vi "SNA Driver Calibration Popup.vi"(8 "error in (no error)":errorcluster, 10 "RequestedCal":string, 11 "Message (\"\")":string) -> (0 "error out":errorcluster)   [LabVIEW 2011]
panel:
  in  "OK":bool
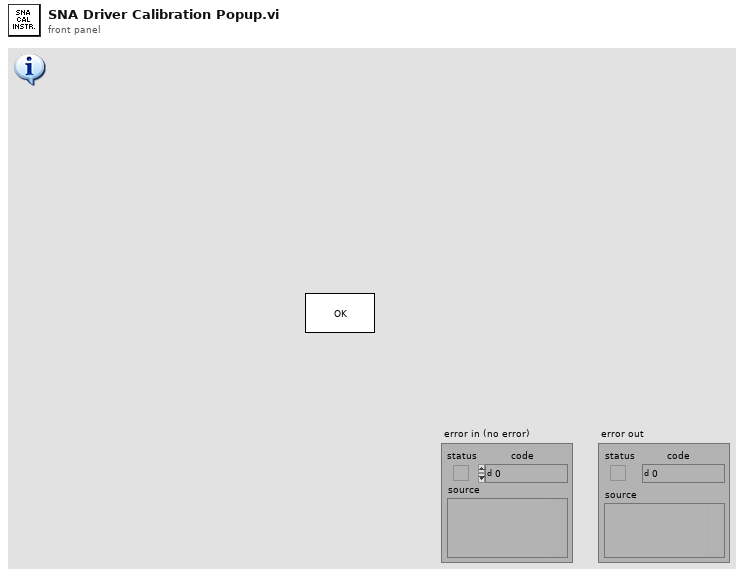
[diagram p1: front panel]
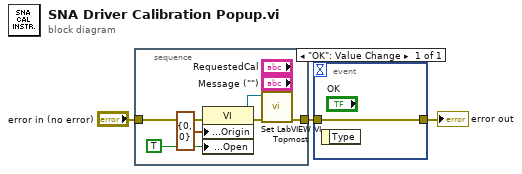
[diagram p0: block diagram]
diagram:
  n1 = stacked-sequence {
    tunnel: "error in (no error)" -> [w9]
    tunnel: [w6] -> w1
    frame #0 {
      n2 = property on="Property Node" class="VI"(error in=w9, "Front Panel Window:Origin"=cluster{"Horizontal":i16, "Vertical":i16} {"Horizontal"=0, "Vertical"=0}, "Front Panel Window:Open"=TRUE) -> (reference out=w5:refnum<vi>, error out=w7:errorcluster)  [unwired: 1 in]
      n3 = call "Set LabVIEW VI Topmost.vi"("error in (no error)"=w7, "VI Refnum (null)"=w5) -> ("error out"=w6:errorcluster)  [unwired: 7 in, 2 out]
    }
  }
  n4 = event shown="[0] \"OK\": Value Change" {
    selector: _ -> [_]
    dyn-events: _ -> [_]
    timeout: _ -> [_]
    tunnel: w1 -> [w10]
    tunnel: [w10] -> w3
    event "OK": Value Change {
      n5 = event-data() -> ()  [unwired: 2 out]
    }
  }
  "error out" <- w3
